vi "PCO_ConvertSetDisplay.vi"(8 "error in (no error)":errorcluster {"code" format="%x"}, 10 "strDisplay":T1, 11 "ph":u64) -> (0 "error out":errorcluster {"code" format="%x"}, 2 "ErrorMessage":i32 format="%x", 3 "ph out":u64)   [LabVIEW 2020, in "Convert.lvlib"]
doc: "int PCOCONVERT_API PCO_ConvertSetDisplay(HANDLE ph, PCO_Display* pstrDisplay);"
uses:
  Convert.lvlib
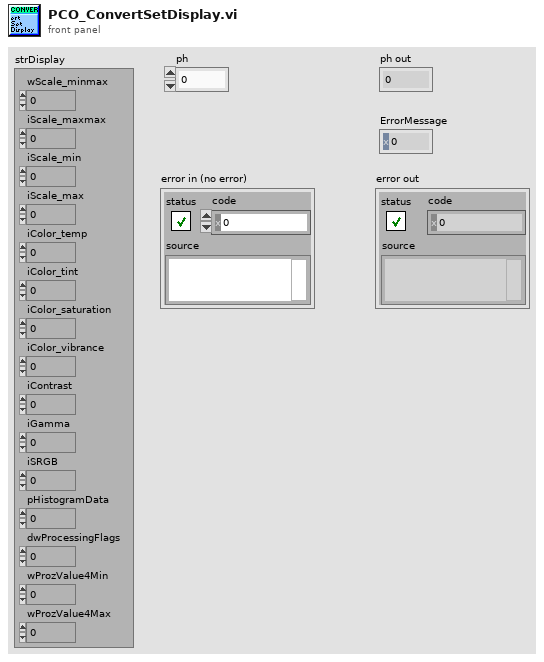
[diagram p1: front panel]
types:
  T1 = cluster{"wScale_minmax":u16, "iScale_maxmax":i32, "iScale_min":i32, "iScale_max":i32, "iColor_temp":i32, "iColor_tint":i32, "iColor_saturation":i32, "iColor_vibrance":i32, "iContrast":i32, "iGamma":i32, "iSRGB":i32, "pHistogramData":u64, "dwProcessingFlags":u32, "wProzValue4Min":u16, "wProzValue4Max":u16}
  T2 = cluster{"wSize":u16, "wScale_minmax":u16, "iScale_maxmax":i32, "iScale_min":i32, "iScale_max":i32, "iColor_temp":i32, "iColor_tint":i32, "iColor_saturation":i32, "iColor_vibrance":i32, "iContrast":i32, "iGamma":i32, "iSRGB":i32, "pHistogramData":u64, "dwDialogOpenFlags":u32, "dwProcessingFlags":u32, "wProzValue4Min":u16, "wProzValue4Max":u16, "dwzzDummy1":cluster{u32, u32, u32, u32, u32, u32, u32, u32, u32, u32, u32, u32, u32, u32, u32, u32, u32, u32, u32, u32, u32, u32, u32, u32, u32, u32, u32, u32, u32, u32, u32, u32, u32, u32, u32, u32, u32, u32, u32, u32, u32, u32, u32, u32, u32, u32, u32, u32, u32, u32}}
  T3 = cluster{"wSize":u16, "wScale_minmax":u16, "iScale_maxmax":i32, "iScale_min":i32, "iScale_max":i32, "iColor_temp":i32, "iColor_tint":i32, "iColor_saturation":i32, "iColor_vibrance":i32, "iContrast":i32, "iGamma":i32, "iSRGB":i32, "pHistogramData":u32, "dwDialogOpenFlags":u32, "dwProcessingFlags":u32, "wProzValue4Min":u16, "wProzValue4Max":u16, "dwzzDummy1":cluster{u32, u32, u32, u32, u32, u32, u32, u32, u32, u32, u32, u32, u32, u32, u32, u32, u32, u32, u32, u32, u32, u32, u32, u32, u32, u32, u32, u32, u32, u32, u32, u32, u32, u32, u32, u32, u32, u32, u32, u32, u32, u32, u32, u32, u32, u32, u32, u32, u32}}
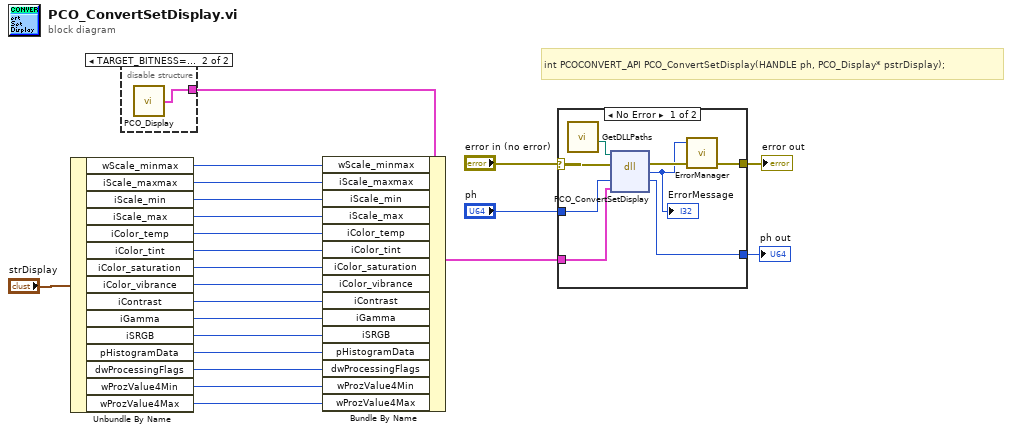
[diagram p0: block diagram]
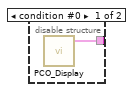
[diagram p2: hidden frame]
diagram:
  # "int PCOCONVERT_API PCO_ConvertSetDisplay(HANDLE ph, PCO_Display* pstrDisplay);"
  n1 = Unbundle By Name("strDisplay") -> ("wScale_minmax"=w18:u16, "iScale_maxmax"=w17:i32, "iScale_min"=w16:i32, "iScale_max"=w15:i32, "iColor_temp"=w14:i32, "iColor_tint"=w13:i32, "iColor_saturation"=w12:i32, "iColor_vibrance"=w11:i32, "iContrast"=w10:i32, "iGamma"=w9:i32, "iSRGB"=w8:i32, "pHistogramData"=w7:u64, "dwProcessingFlags"=w3:u32, "wProzValue4Min"=w2:u16, "wProzValue4Max"=w1:u16)
  n2 = disable-structure "Diagram Disable Structure" shown="TARGET_BITNESS==32" {
    disable-tunnel: [w23 w24] -> w6
    frame condition #0 {
      n3 = call "PCO_Display.vi"() -> ("PCO_DisplayRaw_x64"=w23:T2)  [unwired: 4 in, 4 out]
    }
    frame condition #1 (active) {
      n4 = call "PCO_Display.vi"() -> ("PCO_DisplayRaw_win32"=w24:T3)  [unwired: 4 in, 4 out]
    }
  }
  n5 = Bundle By Name(cluster=w6, "wScale_minmax"=w18, "iScale_maxmax"=w17, "iScale_min"=w16, "iScale_max"=w15, "iColor_temp"=w14, "iColor_tint"=w13, "iColor_saturation"=w12, "iColor_vibrance"=w11, "iContrast"=w10, "iGamma"=w9, "iSRGB"=w8, "pHistogramData"=w7, "dwProcessingFlags"=w3, "wProzValue4Min"=w2, "wProzValue4Max"=w1) -> (w5:T3)
  n6 = case shown="No Error" "error in (no error)" {
    selector: "error in (no error)" -> [w29 w34]
    tunnel: "ph" -> [w32 w33]
    tunnel: [w31 w33] -> w21
    tunnel: w5 -> [w30 _]
    tunnel: [w27 w34] -> w20
    frame No Error {
      n7 = call "GetDLLPaths.vi"() -> ("PCO_Conv_Path"=w25:path)  [unwired: 9 in, 2 out]
      n8 = dll-call lib="?" fn="PCO_ConvertSetDisplay"(path in=w25, error in=w29, "ph"=w32, "pstrDisplay"=w30) -> (error out=w28:errorcluster, "return type"=w26:i32, "ph"=w31:u64)  [unwired: 2 in, 1 out]
      "ErrorMessage" <- w26
      n9 = call "ErrorManager.vi"("error in (no error)"=w28, "error code"=w26) -> ("error out"=w27:errorcluster)  [unwired: 3 in]
    }
    frame Error {
    }
  }
  "ph out" <- w21
  "error out" <- w20
